vi "DAQmx Rollback Channel If Error.vi"(0 "task in":refnum<k21>, 5 "channel names":string, 11 "error in":errorcluster) -> (4 "task out":refnum<k21>, 15 "error out":errorcluster)   [LabVIEW 2011]
uses:
  nilvaiu.dll
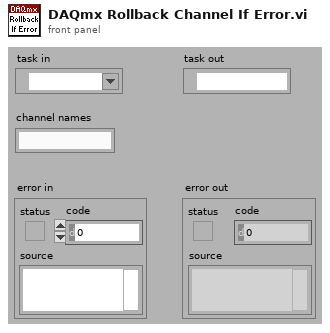
[diagram p1: front panel]
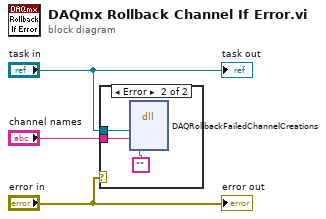
[diagram p0: block diagram]
diagram:
  n1 = case shown="Error" "error in" {
    tunnel: "task in" -> [_ w6]
    tunnel: "channel names" -> [_ w5]
    frame No Error {
    }
    frame Error {
      n2 = dll-call lib="nilvaiu.*" fn="DAQRollbackFailedChannelCreations"("taskID"=w6, "channelNames"=w5, "extendedErrorInfo"="") -> ()  [unwired: 4 in, 5 out]
    }
  }
  "error out" <- "error in"
  "task out" <- "task in"
